vi "rename channel in mapping.vi"(7 "owner ID":string, 8 "error in":errorcluster, 9 "new action channel":refnum<class "TBM channel.lvclass">, 10 "old action channel":refnum<class "TBM channel.lvclass">, 11 "engine configuration in":refnum<class "Simple Sequencer TBM configuration.lvclass">) -> (0 "error out":errorcluster, 3 "engine configuration out":refnum<class "Simple Sequencer TBM configuration.lvclass">)   [LabVIEW 2014, in "Simple Sequencer TBM configuration.lvclass"]
uses:
  <vilib>/NI/TBM Modules/Sequencer/module/configuration/Simple Sequencer TBM configuration.lvclass
  <vilib>/NI/Tag Bus Module Framework/channel/TBM channel.lvclass
  <vilib>/NI/Tag Bus Module Framework/root configuration/TBM configuration.lvclass
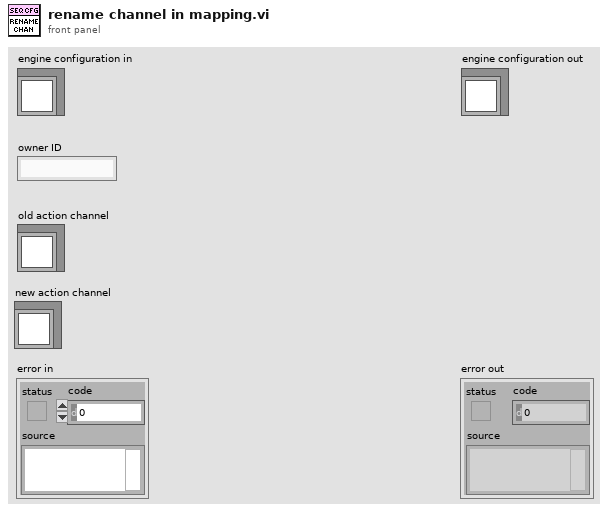
[diagram p1: front panel]
types:
  T1 = typedef "tag bus.lvlib/data table.lvlib/mapping specification.ctl" = cluster{"data type":T2, "mappings":T3[]}
  T2 = typedef "tag bus.lvlib/tag descriptor.lvclass/Data Type.ctl" = enum16{"Double", "Single", "I64", "I32", "I16", "I8", "U64", "U32", "U16", "U8", "Boolean", "String", "Array of Double", "Array of Single", "Array of I64", "Array of I32", "Array of I16", "Array of I8", "Array of U64", "Array of U32", "Array of U16", "Array of U8", "Array of Boolean", "Array of String"}
  T3 = typedef "tag bus.lvlib/data table.lvlib/mapping.ctl" = cluster{"sink name":string, "source name":string}
  T4 = typedef "TBM channel.lvclass/channel classification.ctl" = enum16{"input data", "output data", "processing parameter", "processing result"}
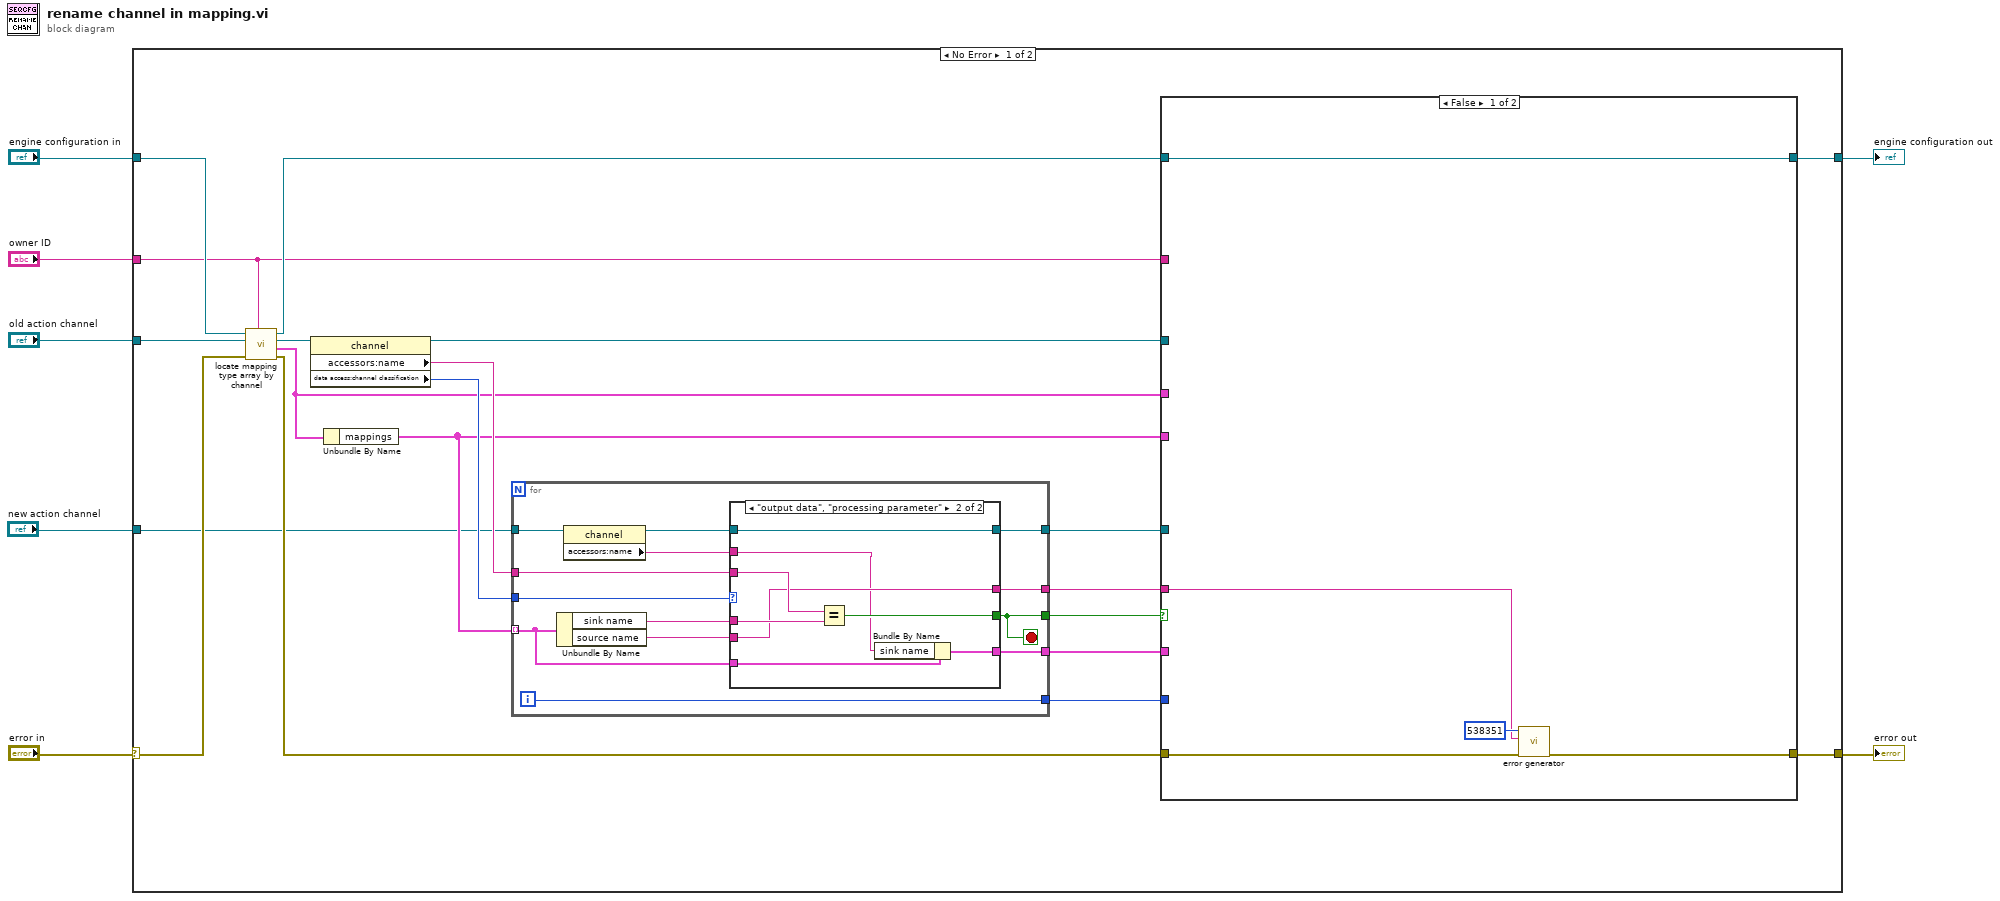
[diagram p0: block diagram]
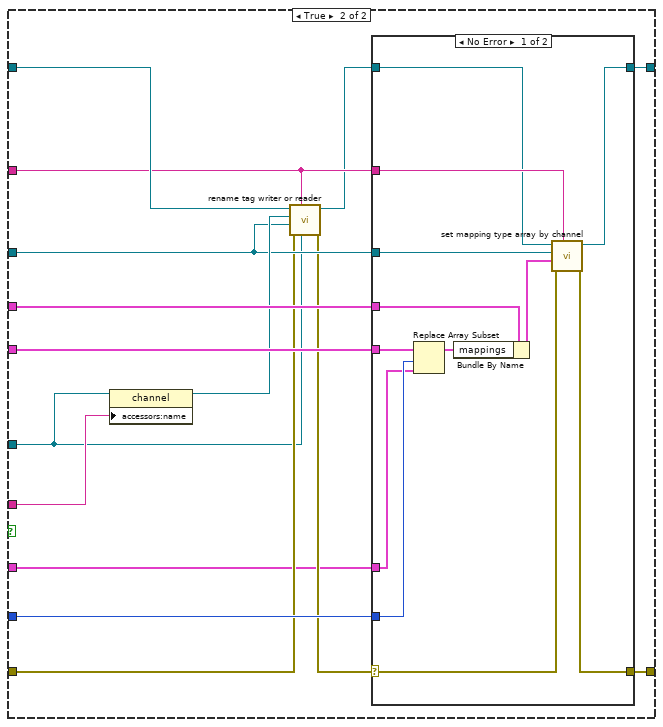
[diagram p2: hidden frame]
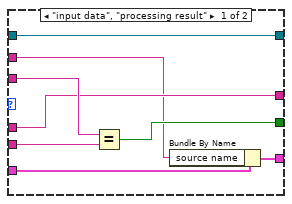
[diagram p4: hidden frame]
diagram:
  n1 = case shown="No Error" "error in" {
    selector: "error in" -> [w16 w92]
    tunnel: [w27 w92] -> w6
    tunnel: [w26 w91] -> w4
    tunnel: "engine configuration in" -> [w19 w91]
    tunnel: "owner ID" -> [w12 _]
    tunnel: "old action channel" -> [w17 _]
    tunnel: "new action channel" -> [w10 _]
    frame No Error {
      n2 = call <vilib>:"locate mapping type array by channel.vi"("owner ID"=w12, "error in"=w16, "channel"=w17, "engine configuration in"=w19) -> ("error out"=w15:errorcluster, "Mapping"=w13:T1, "channel out"=w14:refnum<class "TBM channel.lvclass">, "engine configuration out"=w18:refnum<class "Simple Sequencer TBM configuration.lvclass">)  [unwired: 4 in]
      n3 = property class="channel"(reference=w14) -> (reference out=w20:refnum<class "TBM channel.lvclass">, "accessors:name"=w24:string, "data access:channel classification"=w25:T4)  [unwired: 1 in, 1 out]
      n4 = Unbundle By Name(w13) -> ("mappings"=w21:T3[])
      n5 = for {
        tunnel: w21 -> [w65] mode=indexing
        tunnel: w25 -> [w74]
        tunnel: w24 -> [w71]
        tunnel: [w70] -> w23
        tunnel: [w69] -> w22
        tunnel: [w68] -> w11
        tunnel: w10 -> [w67]
        tunnel: [w64] -> w9
        tunnel: [w62] -> w8
        i -> [w69]
        stop <- w70 stop-if-true
        n6 = Unbundle By Name(w65) -> ("sink name"=w73:string, "source name"=w72:string)
        n7 = property class="channel"(reference=w67) -> (reference out=w63:refnum<class "TBM channel.lvclass">, "accessors:name"=w66:string)  [unwired: 1 in, 1 out]
        n8 = case shown="\"output data\", \"processing parameter\"" w74 {
          tunnel: w73 -> [w79 w89]
          tunnel: w72 -> [w82 w87]
          tunnel: w71 -> [w81 w90]
          tunnel: [w80 w88] -> w70
          tunnel: [w79 w87] -> w68
          tunnel: w66 -> [w78 w85]
          tunnel: w65 -> [w77 w86]
          tunnel: [w76 w84] -> w64
          tunnel: w63 -> [w75 w83]
          tunnel: [w75 w83] -> w62
          frame "input data", "processing result" {
            n9 = Equal?(x=w81, y=w82) -> (x = y?=w80:bool)
            n10 = Bundle By Name(cluster=w77, "source name"=w78) -> (w76:T3)
          }
          frame "output data", "processing parameter" {
            n11 = Equal?(x=w90, y=w89) -> (x = y?=w88:bool)
            n12 = Bundle By Name(cluster=w86, "sink name"=w85) -> (w84:T3)
          }
        }
      }
      n13 = case shown="False" w23 {
        tunnel: w15 -> [w30 w37]
        tunnel: w22 -> [_ w46]
        tunnel: w21 -> [_ w47]
        tunnel: w13 -> [_ w45]
        tunnel: w20 -> [_ w38]
        tunnel: w18 -> [w32 w41]
        tunnel: [w32 w44] -> w26
        tunnel: [w28 w43] -> w27
        tunnel: w12 -> [_ w40]
        tunnel: w11 -> [w29 w42]
        tunnel: w9 -> [_ w34]
        tunnel: w8 -> [_ w33]
        frame False {
          n14 = call <vilib>:"error generator.vi"("error in"=w30, "append error message"=w29, "error code (0)"=538351) -> ("error out"=w28:errorcluster)  [unwired: 6 in]
        }
        frame True {
          n15 = property class="channel"(reference=w33, "accessors:name"=w42) -> (reference out=w39:refnum<class "TBM channel.lvclass">)  [unwired: 1 in, 1 out]
          n16 = call <vilib>:"rename tag writer or reader.vi"("new channel"=w33, "owner ID"=w40, "error in"=w37, "old channel"=w38, "tag descriptor"=w39, "engine configuration in"=w41) -> ("error out"=w36:errorcluster, "engine configuration out"=w35:refnum<class "Simple Sequencer TBM configuration.lvclass">)  [unwired: 4 in]
          n17 = case shown="No Error" w36 {
            selector: w36 -> [w53 w60]
            tunnel: w47 -> [w51 _]
            tunnel: w46 -> [w49 _]
            tunnel: w45 -> [w59 _]
            tunnel: [w57 w61] -> w44
            tunnel: [w56 w60] -> w43
            tunnel: w40 -> [w55 _]
            tunnel: w38 -> [w54 _]
            tunnel: w35 -> [w52 w61]
            tunnel: w34 -> [w48 _]
            frame No Error {
              n18 = Replace Array Subset(array=w51, new element=w48, index=w49) -> (w50:T3[])
              n19 = Bundle By Name(cluster=w59, "mappings"=w50) -> (w58:T1)
              n20 = call <vilib>:"set mapping type array by channel.vi"("owner ID"=w55, "error in"=w53, "Mapping"=w58, "channel"=w54, "engine configuration in"=w52) -> ("error out"=w56:errorcluster, "engine configuration out"=w57:refnum<class "Simple Sequencer TBM configuration.lvclass">)  [unwired: 5 in]
            }
            frame Error {
            }
          }
        }
      }
    }
    frame Error {
    }
  }
  "error out" <- w6
  "engine configuration out" <- w4
